vi "Test 1 Parse Number.vi"(8 "error in (no error)":errorcluster, 11 "Test Case In":refnum<class "Schema parsing test.lvclass">) -> (0 "error out":errorcluster, 3 "Test Case Out":refnum<class "Schema parsing test.lvclass">)   [LabVIEW 2020, in "Schema parsing test.lvclass"]
uses:
  Schema parsing test.lvclass
  C:/Program Files (x86)/National Instruments/LabVIEW 2020/vi.lib/Astemes/LUnit/Test Case.lvclass
  <vilib>/Astemes/LUnit/Test Case.lvclass/Test Case.ctl
  4993e8ee-a06a-463a-9684-69129f64d5ce.vi
  22a963e1-d34d-4fb5-aba3-09113b8ee329.vi
  <vilib>/Astemes/LUnit/Append Pass Result.vi
  <vilib>/Astemes/LUnit/Append Fail Result.vi
  <vilib>/Astemes/LUnit/Describe Comparison.vi
  <vilib>/Astemes/LUnit/Compare Variants.vi
  <vilib>/Astemes/LUnit/Variant to string.vi
  <vilib>/Utility/Data Type/Get Type Information.vi
  <vilib>/Utility/LVClass/Get LV Class Name.vi
  Number/Number.lvclass
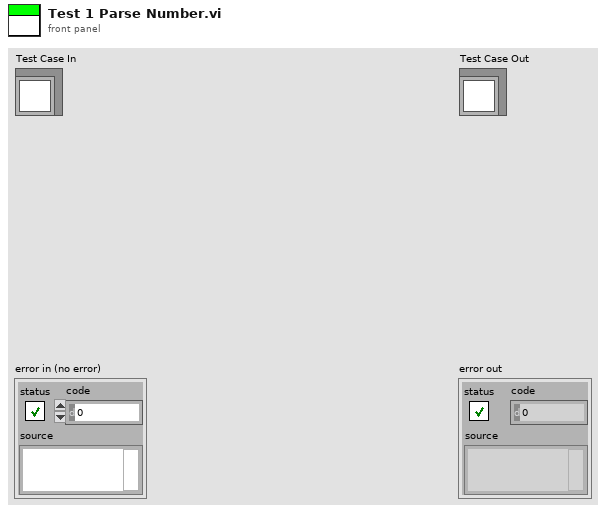
[diagram p1: front panel]
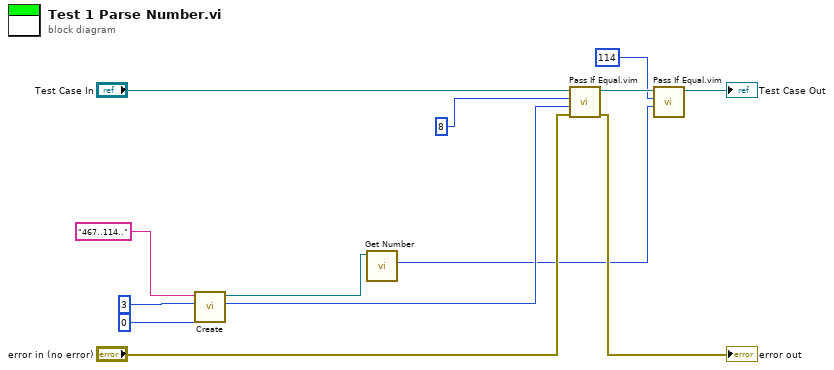
[diagram p0: block diagram]
diagram:
  n1 = call "Create.vi"("Row"=0, "Col Offset"=3, "String"="467..114..") -> ("Offset Past Number"=w5:i32, "Number"=w4:refnum<class "Number.lvclass">)  [unwired: 6 in, 1 out]
  n2 = call "Get Number.vi"("Number in"=w4) -> ("Number"=w2:i32)  [unwired: 8 in, 2 out]
  n3 = call "Pass If Equal.vim"("error in (no error)"="error in (no error)", "Actual"=w5, "Expected"=8 ("Col"), "LUnit Test Case In"="Test Case In") -> ("error out"=→"error out":errorcluster, "LUnit Test Case Out"=w12:refnum<class "Schema parsing test.lvclass">)  [unwired: 6 in]
  n4 = call "Pass If Equal.vim"("Actual"=w2, "Expected"=114 ("Number"), "LUnit Test Case In"=w12) -> ("LUnit Test Case Out"=→"Test Case Out":refnum<class "Schema parsing test.lvclass">)  [unwired: 7 in, 1 out]
